vi "LCDExample.vi"() -> ()   [LabVIEW 2013]
panel:
  in  "Line 2":string
  in  "Line 1":string
  out "error out":errorcluster
  in  "Baud Rate":u32=9600
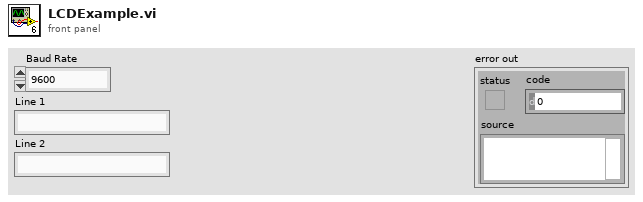
[diagram p1: front panel]
types:
  T1 = typedef "LCDRef.ctl" = cluster{"SerialPortRef":T2}
  T2 = typedef "WPI_SerialPortRef.ctl" = cluster{"DevStatus":errorcluster, "Serial Port Name":refnum<visa-resource-name>}
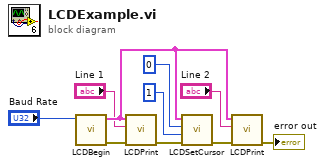
[diagram p0: block diagram]
diagram:
  n1 = call "LCDBegin.vi"("Baud Rate"="Baud Rate") -> ("error out"=w8:errorcluster, "LCDRef"=w9:T1)  [unwired: 9 in]
  n2 = call "LCDPrint.vi"("error in (no error)"=w8, "TextToWrite"="Line 1", "LCDRef"=w9) -> ("error out"=w7:errorcluster)  [unwired: 8 in]
  n3 = call "LCDSetCursor.vi"("error in (no error)"=w7, "Row"=u8 1, "Col"=u8 0, "LCDRef"=w9) -> ("error out"=w6:errorcluster)  [unwired: 7 in]
  n4 = call "LCDPrint.vi"("error in (no error)"=w6, "TextToWrite"="Line 2", "LCDRef"=w9) -> ("error out"=→"error out":errorcluster)  [unwired: 8 in]
